vi "Translate gRPC Method FullName.vi"(8 "error in (no error)":errorcluster, 11 "Method Full Name in":string) -> (0 "error out":errorcluster, 3 "Method Full Name out":string)   [LabVIEW 2019, in "gRPC Scripting Tools.lvlib"]
uses:
  gRPC Scripting Tools.lvlib
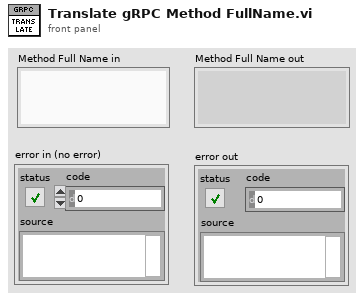
[diagram p1: front panel]
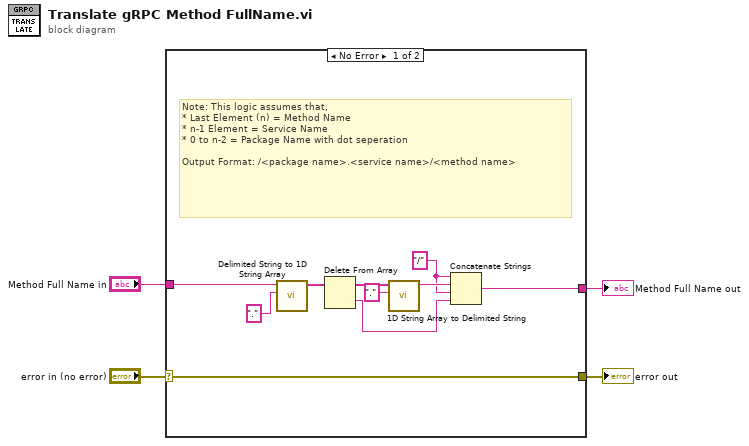
[diagram p0: block diagram]
diagram:
  n1 = case shown="No Error" "error in (no error)" {
    selector: "error in (no error)" -> [w11 w16]
    tunnel: [w10 w15] -> w4
    tunnel: "Method Full Name in" -> [w13 w15]
    tunnel: [w11 w16] -> w1
    frame No Error {
      w6 = "/"
      # "Note: This logic assumes that,\n* Last Element (n) = Method Name\n* n-1 Element = Service Name\n* 0 to n-2 = Package Name with dot seperation\n\nOutput Format: /<package name>.<service name>/<method name>"
      n2 = call <vilib>:"Delimited String to 1D String Array.vi"("delimiter"=".", "delimited string"=w13) -> ("string array"=w14:string[])  [unwired: 9 in]
      n3 = Delete From Array(array=w14) -> (deleted portion=w5:string, array with subset deleted=w9:string[])  [unwired: 2 in]
      n4 = call <vilib>:"1D String Array to Delimited String.vi"("delimiter"=".", "string array"=w9) -> ("delimited string"=w7:string)  [unwired: 9 in]
      n5 = Concatenate Strings(w6, w7, w6, w5) -> (w10:string)
    }
    frame Error {
    }
  }
  "Method Full Name out" <- w4
  "error out" <- w1
